vi "SetHovaCAL_MFC_Concentration.vi"(8 "error in (no error)":errorcluster caption="Fehler (Eingang, kein Fehler)") -> (0 "error out":errorcluster caption="Fehler (Ausgang)")   [LabVIEW 2020, in "Linearisierung v2.lvlib" / "SpanEinstellungen.lvlib"]
uses:
  SpanEinstellungen.lvlib
  Gasteiler/Aktionen FGV Gasteiler Daten.ctl
  GasteilerType.ctl
  Gasteiler/HovaCAL_Interface/Kommunikation/Aktion FGV HovaCAL Interface Autolin.ctl
  Gasteiler/HovaCal/Aktion_FGV_Betriebsdaten.ctl
  Gasteiler/HovaCal/HovaCal.lvlib
  Gasteiler/HovaCAL_Interface/Kommunikation/Kommunikation.lvlib
  Gasteiler/Gasteiler.lvlib
  Linearisierung v2.lvlib
  Gasteiler/HovaCAL_Interface/Helper/Helper.lvlib
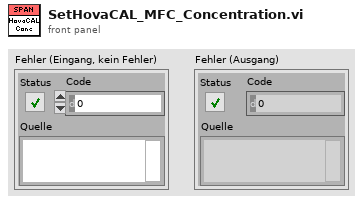
[diagram p1: front panel]
types:
  T1 = typedef "Linearisierung v2.lvlib/GasteilerType.ctl" = u16
  T2 = typedef "Linearisierung v2.lvlib/Gasteiler.lvlib/Aktionen FGV Gasteiler Daten.ctl" = enum16{"lesen", "Gasteiler Daten", "Seriellen Param.", "MB-Endwert", "laden", "speichern", "Anforderung", "TCP", "Aufzeichnung Start"}
  T3 = typedef "Linearisierung v2.lvlib/Gasteiler.lvlib/Gasteiler Daten.ctl" = cluster{"Gasteiler":T4, "Gasteiler Stufen":T5, "Gasteiler Type":T1, "Konfig Gasteiler":T6, "Gasteiler Span Eingänge":u16}
  T4 = typedef "String - Eingabefeld.ctl" = string
  T5 = typedef "Linearisierung v2.lvlib/Gasteiler.lvlib/Gasteiler Stufen.ctl" = u16
  T6 = typedef "System Einstellungen V2.lvlib/Gasteiler Auswahl.ctl" = u16
  T7 = typedef "Linearisierung v2.lvlib/Gasteiler.lvlib/HovaCAL_Interface.lvlib/Kommunikation.lvlib/Aktion FGV HovaCAL Interface Autolin.ctl" = enum16{"lesen", "schreiben", "MFC Komponente fix setzen", "init"}
  T8 = typedef "Linearisierung v2.lvlib/Gasteiler.lvlib/HovaCal.lvlib/Aktion_FGV_Betriebsdaten.ctl" = enum16{"Lesen", "Sollwerte schreiben", "Sollwerte lesen", "Gase schreiben", "Gase lesen", "Dynamische Werte", "GaseRef", "Gase aendern"}
  T9 = typedef "Auswahlfeld.ctl" = u16
  T10 = typedef "String - Ausgabefeld.ctl" = string
  T11 = typedef "Linearisierung v2.lvlib/Gasteiler.lvlib/HovaCal.lvlib/Betriebsdaten.ctl" = cluster{"Gesamtdurchfluss":dbl, "Eingangskonzentration \nTrägergas":dbl, "Eingangskonzentration\nKomponente 1":dbl, "Eingangskonzentration \nKomponente 2":dbl, "Ausgangskonzentration \nKomponente 1 ":dbl, "Ausgangskonzentration\nKomponente 2":dbl, "l/min -> ml/min":bool, "N2 %->ppm":bool, "Komp1 ppm->%":bool, "Komp2ppm->%":bool, "Sollkomp1ppm->%":bool, "Sollkomp2ppm->%":bool}
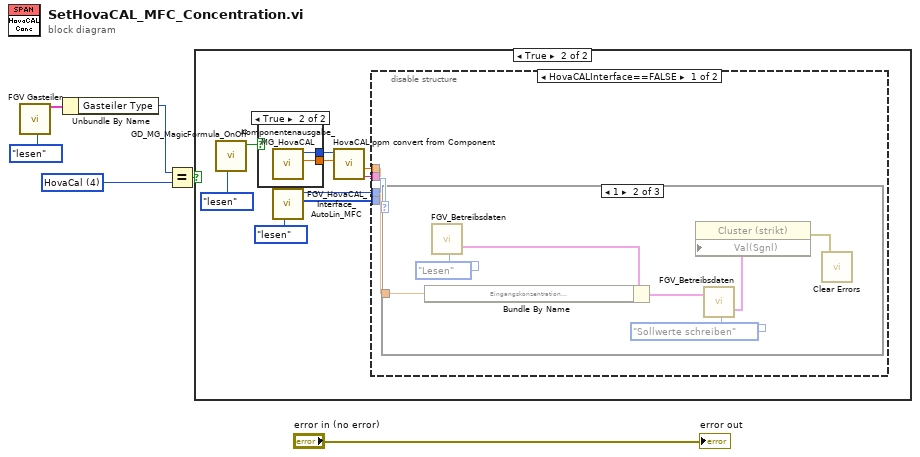
[diagram p0: block diagram]
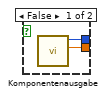
[diagram p3: hidden frame]
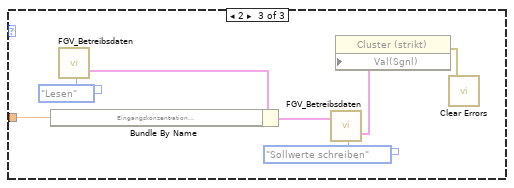
[diagram p5: hidden frame]
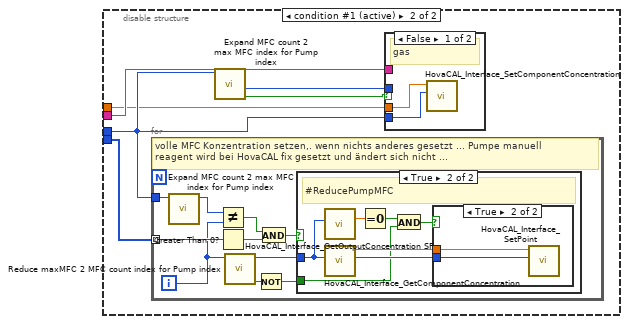
[diagram p6: hidden frame]
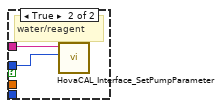
[diagram p7: hidden frame]
diagram:
  w3 = T1 4 items=["LCD-Touch-Display", "Analog-Display", "AVL GDU", "Horiba GDC", "HovaCal", "Horiba 710 c"] ("x")
  n1 = call "FGV Gasteiler.vi"("Aktionen"=Aktionen_FGV_Gasteiler_Daten."lesen") -> ("Gasteiler Daten"=w4:T3)  [unwired: 11 in, 7 out]
  n2 = Unbundle By Name(w4) -> ("Gasteiler Type"=w2:T1)
  n3 = Equal?(x=w2, y=w3) -> (x = y?=w1:bool)
  n4 = case shown="True" w1 {
    frame False {
    }
    frame True {
      n5 = call "GD_MG_MagicFormula_OnOff.vi"("Aktion"=enum16{"lesen", "schreiben", "init"}."lesen") -> ("MG_use_magic_formula"=w8:bool)  [unwired: 8 in, 1 out]
      n6 = case shown="True" w8 {
        tunnel: [w17 w19] -> w10
        tunnel: [w16 w18] -> w9
        frame False {
          n7 = call "Komponentenausgabe.vi"() -> ("Konzentration"=w16:sgl, "Gaskomponente"=w17:T9)  [unwired: 8 in, 2 out]
        }
        frame True {
          n8 = call "Komponentenausgabe_MG_HovaCAL.vi"() -> ("GesamtKonzentration"=w18:sgl, "Gaskomponente"=w19:T9)  [unwired: 3 in, 7 out]
        }
      }
      n9 = call "FGV_HovaCAL_Interface_AutoLin_MFC.vi"("Aktion"=Aktion_FGV_HovaCAL_Interface_Autolin."lesen") -> ("MFV Komponente fix out"=w13:u16[], "AutoLin MFC out"=w14:u16)  [unwired: 7 in, 2 out]
      n10 = call "HovaCAL ppm convert from Component.vi"("Konzentration"=w9, "Gasnummer"=w10) -> ("Komponenten Name"=w11:T10, "Konzentration in ppm"=w12:dbl)  [unwired: 5 in, 3 out]
      n11 = disable-structure shown="HovaCALInterface==FALSE" {
        disable-tunnel: w14 -> [w21 w37]
        disable-tunnel: w13 -> [_ w41]
        disable-tunnel: w12 -> [w20 w36]
        disable-tunnel: w11 -> [_ w40]
        frame condition #0 {
          n12 = case shown="1" w21 {
            tunnel: w20 -> [_ w26 w33]
            frame 0, Default {
            }
            frame 1 {
              n13 = call "FGV_Betreibsdaten.vi"("Enum"=Aktion_FGV_Betriebsdaten."Lesen" ("Aktion")) -> ("Sollwert für Vergleich"=w24:T11)  [unwired: 11 in, 7 out]
              n14 = Bundle By Name(cluster=w24, "Eingangskonzentration\nKomponente 1"=w26) -> (w28:T11)
              n15 = call "FGV_Betreibsdaten.vi"("Sollwert schreiben"=w28, "Enum"=Aktion_FGV_Betriebsdaten."Sollwerte schreiben" ("Aktion")) -> ("Sollwert für Vergleich"=w25:T11)  [unwired: 10 in, 7 out]
              n16 = property on="Eigenschaftsknoten" class="Cluster (strikt)"("Val(Sgnl)"=w25) -> (error out=w27:errorcluster)  [unwired: 2 in, 1 out]
              n17 = call <vilib>:"Clear Errors.vi"("error in (no error)"=w27) -> ()  [unwired: 5 in, 2 out]
            }
            frame 2 {
              n18 = call "FGV_Betreibsdaten.vi"("Enum"=Aktion_FGV_Betriebsdaten."Lesen" ("Aktion")) -> ("Sollwert für Vergleich"=w31:T11)  [unwired: 11 in, 7 out]
              n19 = Bundle By Name(cluster=w31, "Eingangskonzentration \nKomponente 2"=w33) -> (w35:T11)
              n20 = call "FGV_Betreibsdaten.vi"("Sollwert schreiben"=w35, "Enum"=Aktion_FGV_Betriebsdaten."Sollwerte schreiben" ("Aktion")) -> ("Sollwert für Vergleich"=w32:T11)  [unwired: 10 in, 7 out]
              n21 = property on="Eigenschaftsknoten" class="Cluster (strikt)"("Val(Sgnl)"=w32) -> (error out=w34:errorcluster)  [unwired: 2 in, 1 out]
              n22 = call <vilib>:"Clear Errors.vi"("error in (no error)"=w34) -> ()  [unwired: 5 in, 2 out]
            }
          }
        }
        frame condition #1 (active) {
          n23 = for {
            tunnel: w41 -> [w55] mode=indexing
            tunnel: w37 -> [w49]
            i -> [w51]
            # "volle MFC Konzentration setzen,. wenn nichts anderes gesetzt ... Pumpe manuell\nreagent wird bei HovaCAL fix gesetzt und ändert sich nicht ..."
            n24 = call "Expand MFC count 2 max MFC index for Pump index.vi"("AutoLin MFC"=w49) -> ("MFC idx"=w48:i32)  [unwired: 8 in, 2 out]
            n25 = Not Equal?(x=w48, y=w51) -> (x != y?=w52:bool)
            n26 = Greater Than 0?(x=w55) -> (x > 0?=w54:bool)
            n27 = call "Reduce maxMFC 2 MFC count index for Pump index.vi"("MFC idx"=w51) -> ("Pump"=w47:bool, "AutoLin MFC"=w50:i32)  [unwired: 8 in, 1 out]
            n28 = Not(x=w47) -> (.not. x?=w46:bool)
            n29 = And(x=w52, y=w54) -> (x .and. y?=w53:bool)
            n30 = case shown="True" w53 {
              tunnel: w50 -> [_ w60]
              tunnel: w46 -> [_ w56]
              frame False {
              }
              frame True {
                # "#ReducePumpMFC"
                n31 = call "HovaCAL_Interface_GetOutputConcentration SP.vi"("AutoLin MFC Index"=w60) -> ("Konzentration"=w59:dbl)  [unwired: 8 in, 2 out]
                n32 = call "HovaCAL_Interface_GetComponentConcentration.vi"("AutoLin MFV Index"=w60) -> ("AutoLin MFV Index out"=w62:u32, "Konzentration"=w61:dbl)  [unwired: 8 in, 1 out]
                n33 = Equal To 0?(x=w59) -> (x = 0?=w58:bool)
                n34 = And(x=w58, y=w56) -> (x .and. y?=w57:bool)
                n35 = case shown="True" w57 {
                  tunnel: w62 -> [_ w64]
                  tunnel: w61 -> [_ w63]
                  frame False {
                  }
                  frame True {
                    n36 = call "HovaCAL_Interface_SetPoint.vi"("AutoLin MFC Index"=w64, "Konzentration"=w63) -> ()  [unwired: 9 in, 1 out]
                  }
                }
              }
            }
          }
          n37 = call "Expand MFC count 2 max MFC index for Pump index.vi"("AutoLin MFC"=w37) -> ("Pump"=w39:bool, "Pump Idx"=w38:i32)  [unwired: 8 in, 1 out]
          n38 = case shown="False" w39 {
            tunnel: w40 -> [_ w45]
            tunnel: w38 -> [_ w44]
            tunnel: w37 -> [w43 _]
            tunnel: w36 -> [w42 _]
            frame False {
              # "gas"
              n39 = call "HovaCAL_Interface_SetComponentConcentration.vi"("AutoLin MFV Index"=w43, "Konzentration"=w42) -> ()  [unwired: 7 in, 3 out]
            }
            frame True {
              # "water/reagent"
              n40 = call "HovaCAL_Interface_SetPumpParameter.vi"("Pump Idx"=w44, "Komponent Name"=w45) -> ()  [unwired: 9 in, 1 out]
            }
          }
        }
      }
    }
  }
  "error out" <- "error in (no error)"
